vi "CANOpen Change ID.vi"(8 "error in (no error)":errorcluster, 10 "Node ID":u8 max=127 step=1, 11 "Node Ptr":u64 format="%.0x") -> (0 "error out":errorcluster, 3 "Passed?":bool)   [LabVIEW 2013]
uses:
  Shared Code/CANOpen Addon GUID Lookup Global.vi
  <vilib>/NI Veristand/Custom Device API/Custom Device API.lvlib
  CANOpen Addon Custom Device.lvlib
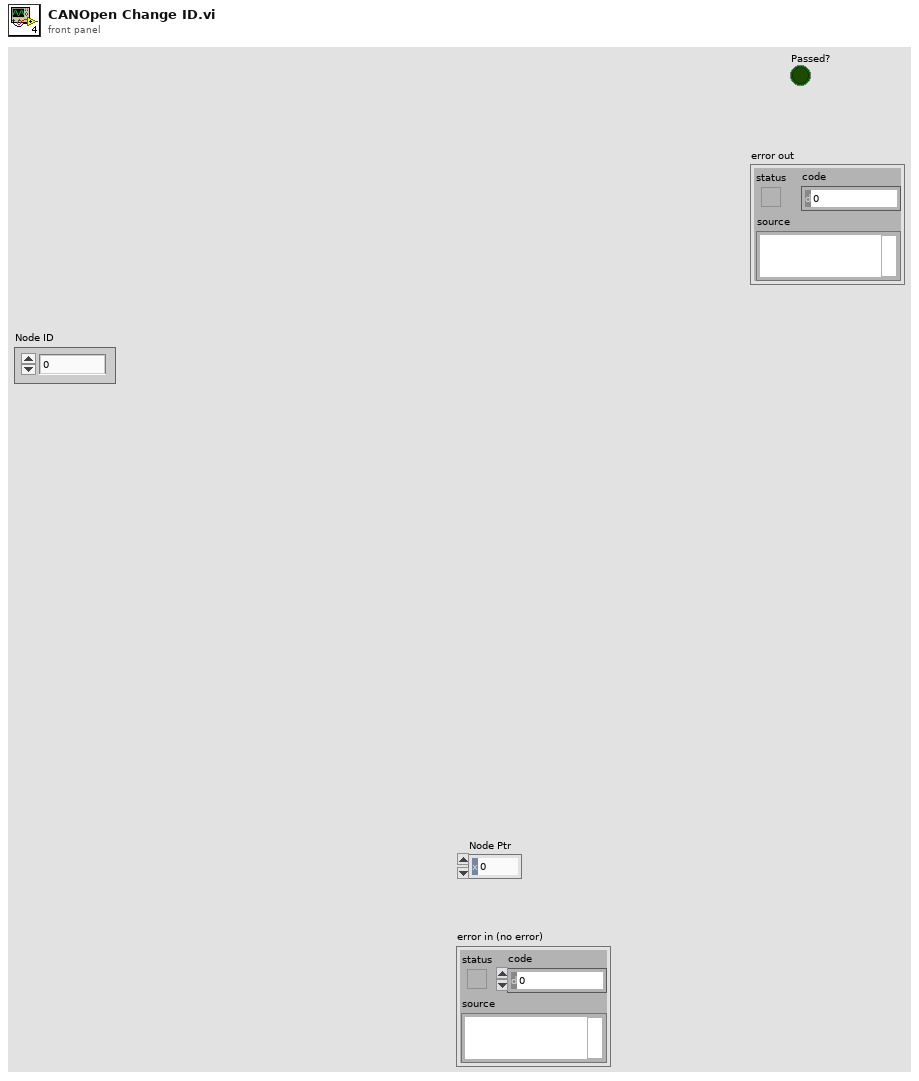
[diagram p1: front panel]
types:
  T1 = typedef "Custom Device API.lvlib/Custom Device Item Ref.ctl" = u64
  T2 = typedef "Custom Device API.lvlib/Custom Device Item Info.ctl" = cluster{"Name":string, "Is Channel":bool, "GUID":string, "Is Waveform":bool}
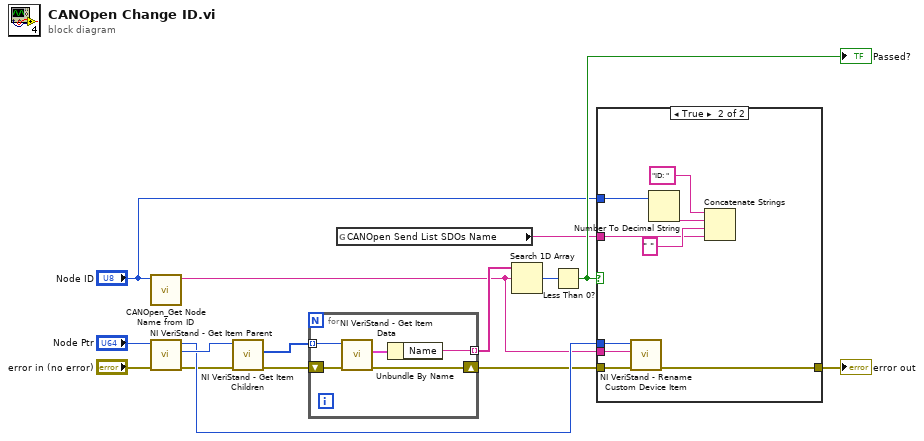
[diagram p0: block diagram]
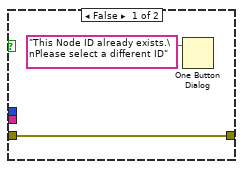
[diagram p2: hidden frame]
diagram:
  n1 = call "CANOpen_Get Node Name from ID.vi"("Node ID"="Node ID") -> ("Node ID Name"=w4:string)  [unwired: 10 in]
  n2 = call <vilib>:"NI VeriStand - Get Item Parent.vi"("error in (no error)"="error in (no error)", "Item Ref in"="Node Ptr") -> ("error out"=w5:errorcluster, "Parent Ref"=w9:T1, "Item Ref out"=w7:T1)  [unwired: 6 in, 1 out]
  n3 = call <vilib>:"NI VeriStand - Get Item Children.vi"("error in (no error)"=w5, "Item Ref in"=w9) -> ("error out"=w15:errorcluster, "Child Refs"=w14:T1[])  [unwired: 6 in, 2 out]
  n4 = for {
    tunnel: w14 -> [w19] mode=indexing
    tunnel: [w16] -> w10 mode=indexing
    shift-right: [w17] -> w3
    shift-left: w15 -> [w18]
    n5 = call <vilib>:"NI VeriStand - Get Item Data.vi"("error in (no error)"=w18, "Item Ref in"=w19) -> ("error out"=w17:errorcluster, "Item Info"=w20:T2)  [unwired: 6 in, 2 out]
    n6 = Unbundle By Name(w20) -> ("Name"=w16:string)
  }
  n7 = global read "CANOpen Addon GUID Lookup Global.vi" "CANOpen Send List SDOs Name"() -> (w1:string)
  n8 = Search 1D Array(1D array=w10, element=w4) -> (index of element=w11:i32)  [unwired: 1 in]
  n9 = Less Than 0?(x=w11) -> (x < 0?=w12:bool)
  "Passed?" <- w12
  n10 = case shown="True" w12 {
    tunnel: [w21 w23] -> w8
    tunnel: w4 -> [_ w31]
    tunnel: w7 -> [_ w30]
    tunnel: w3 -> [w21 w29]
    tunnel: "Node ID" -> [_ w25]
    tunnel: w1 -> [_ w24]
    frame False {
      n11 = One Button Dialog(message="This Node ID already exists.\nPlease select a different ID") -> ()  [unwired: 1 in, 1 out]
    }
    frame True {
      n12 = call <vilib>:"NI VeriStand - Rename Custom Device Item.vi"("error in (no error)"=w29, "New Name"=w31, "Item Ref in"=w30) -> ("error out"=w23:errorcluster)  [unwired: 1 in, 7 out]
      n13 = Number To Decimal String(number=w25) -> (decimal integer string=w27:string)  [unwired: 1 in]
      n14 = Concatenate Strings("ID: " ("string"), w27, " " ("string"), w24) -> ()  [unwired: 1 out]
    }
  }
  "error out" <- w8
